vi "Launch Prefs Session.vi"() -> (0 "error out":errorcluster, 3 "PrefsDB":refnum<class "PrefsDB.lvclass">)   [LabVIEW 2020, in "User Prefs.lvlib" / "PrefsDB.lvclass"]
uses:
  PrefsDB.lvclass
  C:/dev/lv20CE/relink/lv-promises/Promises/Value/Value.lvclass
  lv-promises/Promises/Promise/Promise.lvclass/Promise.ctl
  lv-promises/Promises/Future/Future.lvclass/Future.ctl
  Session Async.vi
  lv-promises/Promises/Future/Future.lvclass
  PrefsDB.lvclass/PrefsDB.ctl
  lv-exec-anchor/ExecAnchor/ExecAnchor.lvclass
  lv-promises/Promises/Promise/Promise.lvclass
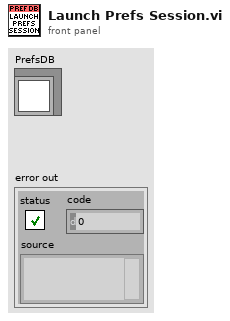
[diagram p1: front panel]
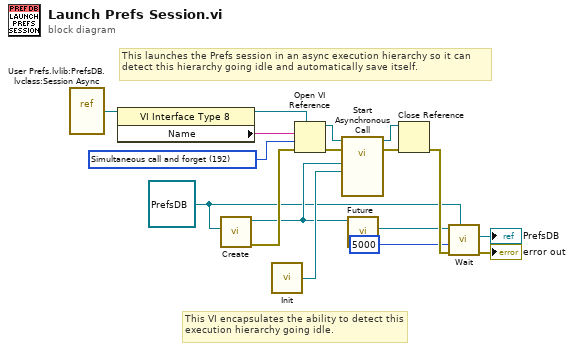
[diagram p0: block diagram]
diagram:
  w4 = refnum<class "PrefsDB.lvclass"> refnum ("User Prefs.lvlib:PrefsDB.lvclass")
  w10 = 192 items=["Record modifications"=1, "Open templates for editing"=2, "Prompt user to save"=4, "Prepare for reentrant run"=8, "Prompt to find missing subVIs"=16, "Hide loading dialog box"=32, "Enable simultaneous calls"=64, "Prepare to call and forget"=128, "Simultaneous call and forget"=192, "Prepare to call and collect"=256, "Simultaneous call and collect"=320]
  # "This VI encapsulates the ability to detect this execution hierarchy going idle."
  # "This launches the Prefs session in an async execution hierarchy so it can detect this hierarchy going idle and automatically save itself."
  n1 = vi-ref "User Prefs.lvlib:PrefsDB.lvclass:Session Async.vi"() -> (w8:refnum<vi>)
  n2 = property class="VI Interface Type 8"(reference=w8) -> (reference out=w11:refnum<vi>, "Name"=w9:string)  [unwired: 1 in, 1 out]
  n3 = call "Create.vi"("Result Type"=w4) -> ("error out"=w16:errorcluster, "Promise"=w6:refnum<class "Promise.lvclass">)  [unwired: 9 in]
  n4 = call "Init.vi"() -> ("ExecAnchor out"=w7:refnum<class "ExecAnchor.lvclass">)  [unwired: 7 in]
  n5 = Open VI Reference(type specifier VI Refnum (for type only)=w11, vi path=w9, options=w10, error in (no error)=w16) -> (vi reference=w13:refnum<vi>, error out=w12:errorcluster)  [unwired: 2 in]
  n6 = call-by-ref "Start Asynchronous Call"(reference=w13, error in=w12, "ExecAnchor"=w7, "Promise"=w6) -> (reference out=w15:refnum<vi>, error out=w14:errorcluster)  [unwired: 10 in]
  n7 = call "Future.vi"("Promise in"=w6) -> ("Future"=w5:refnum<class "Future.lvclass">)  [unwired: 9 in, 1 out]
  n8 = Close Reference(reference=w15, error in (no error)=w14) -> (error out=w17:errorcluster)
  n9 = call "Wait.vi"("Result Type"=w4, "error in (no error)"=w17, "Timeout mS (-1)"=5000, "Future in"=w5) -> ("error out"=→"error out":errorcluster, "Result"=→"PrefsDB":refnum<class "PrefsDB.lvclass">)  [unwired: 6 in]
